vi "OneSensorMagazineLogic.vi"(5 "Intake Side Sensor":bool, 6 "Outtake Button":bool, 7 "Intake Toggle":bool) -> (0 "Intake Pistons":bool, 1 "Kicker Motors":dbl, 2 "Magazine Motors":dbl, 3 "Intake Motors":dbl)   [LabVIEW 2020]
uses:
  MagazineControl.ctl
  OneSensorMagazineLogic.ctl
  TitanLib/Lib/TitanLib.lvlib
panel:
  in  "Initial State":T1
  out "Current State":T2
  in  "Kicker Power":dbl=0.5
  in  "Magazine Power":dbl=1.0
  in  "Input Power":dbl=1.0
  # "Inputs"
  # "Power Levels"
  # "Outputs"
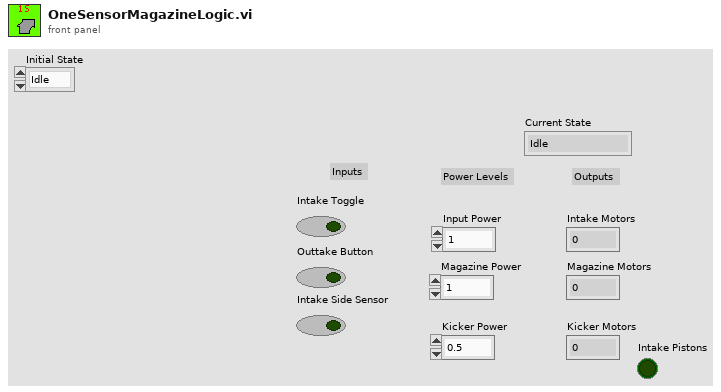
[diagram p1: front panel]
types:
  T1 = typedef "OneSensorMagazineLogic.ctl" = enum16{"Idle", "Intaking", "One Ball", "One Ball Intake", "Two Balls", "Outtake"}
  T2 = typedef "MagazineControl.ctl" = enum16{"Idle", "Intaking", "Outtake", "One Ball", "One Ball Intake", "One Ball Outtake", "Two Balls", "Two Ball Outtake"}
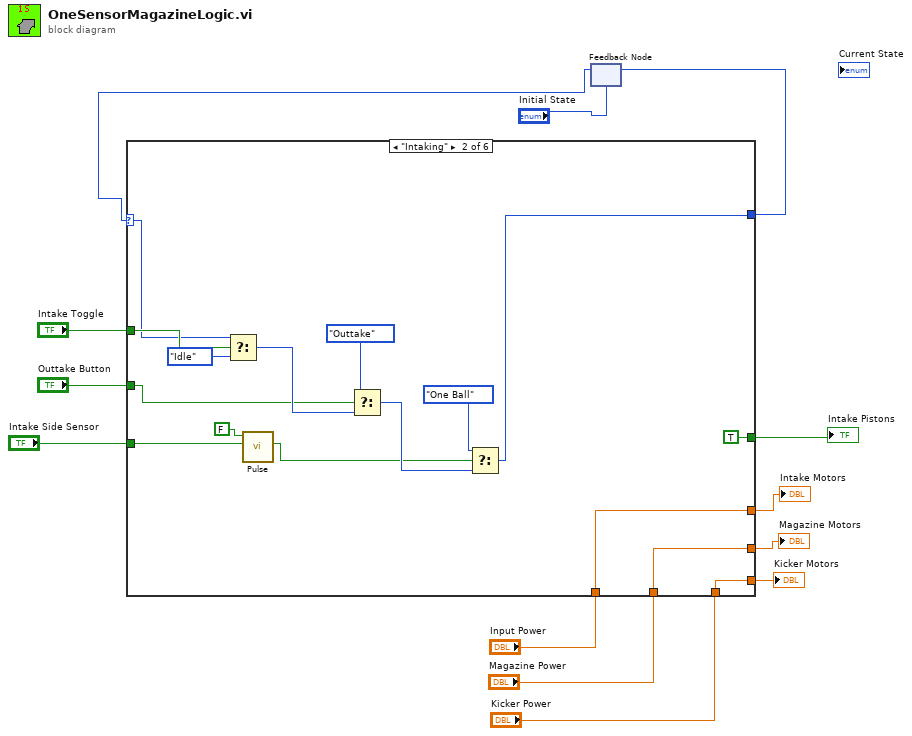
[diagram p0: block diagram]
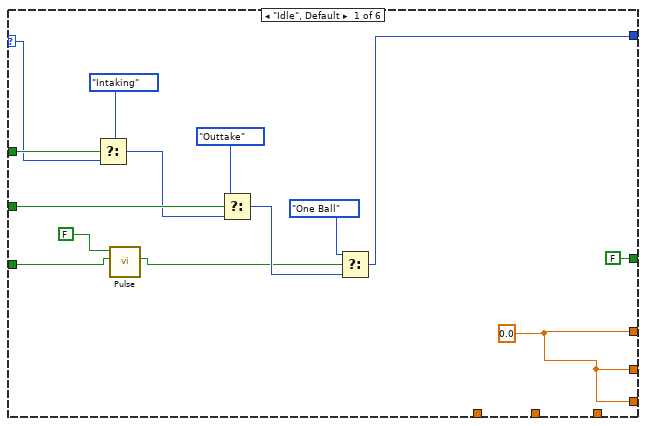
[diagram p2: hidden frame]
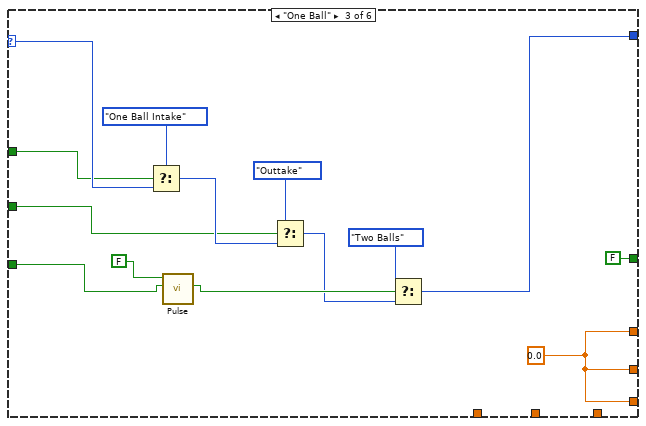
[diagram p3: hidden frame]
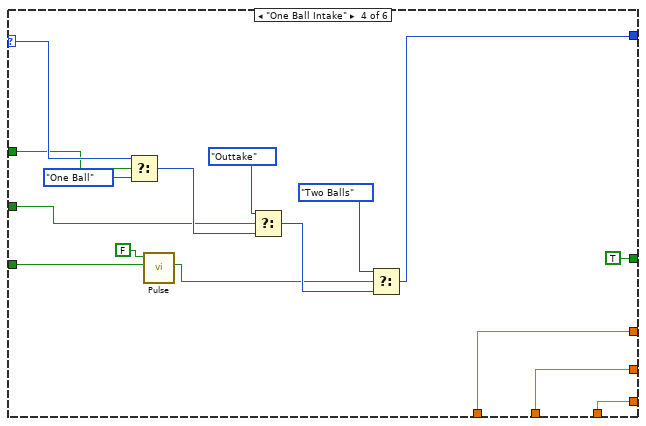
[diagram p4: hidden frame]
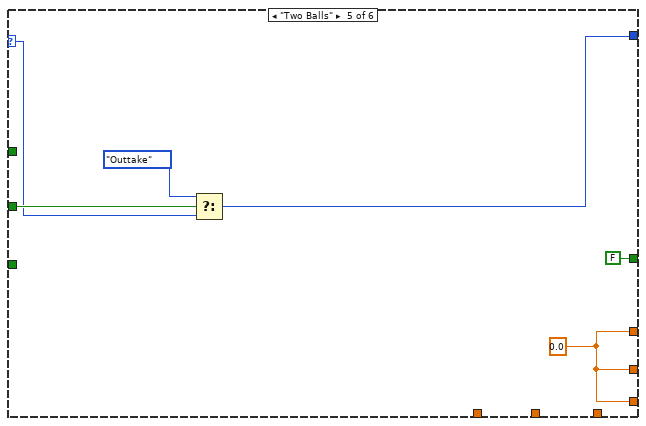
[diagram p5: hidden frame]
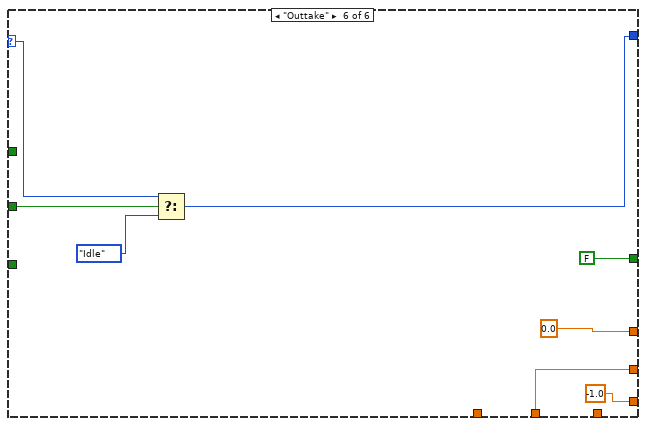
[diagram p6: hidden frame]
diagram:
  n1 = feedback #1("Initial State") -> (w2:T1)
  n2 = case shown="\"Intaking\"" w2 {
    selector: w2 -> [w18 w39 w51 w67 w78 w82]
    tunnel: "Intake Toggle" -> [w27 w41 w50 w66 _ _]
    tunnel: "Outtake Button" -> [w26 w40 w52 w68 w79 w87]
    tunnel: "Intake Side Sensor" -> [w22 w35 w53 w69 _ _]
    tunnel: [w20 w38 w49 w65 w77 0.0 ("Input Power")] -> w8
    tunnel: "Input Power" -> [_ w38 _ w65 _ _]
    tunnel: [w20 w37 w49 w64 w77 w84] -> w10
    tunnel: "Magazine Power" -> [_ w37 _ w64 _ w84]
    tunnel: [w20 w33 w49 w63 w77 -1.0 ("Kicker Motors")] -> w12
    tunnel: "Kicker Power" -> [_ w33 _ w63 _ _]
    tunnel: [FALSE ("Intake Pistons") TRUE ("Intake Pistons") FALSE ("Intake Pistons") TRUE ("Intake Pistons") FALSE ("Intake Pistons") FALSE ("Intake Pistons")] -> w4
    tunnel: [w14 w28 w44 w61 w75 w80] -> w1
    frame "Idle", Default {
      w20 = 0.0 ("Input Power")
      n3 = Select(t=OneSensorMagazineLogic."Intaking", s=w27, f=w18) -> (s? t:f=w25:T1)
      n4 = call "Pulse.vi"("Input"=w22, "Rising Edge?"=FALSE) -> ("Output"=w23:bool)  [unwired: 9 in]
      n5 = Select(t=OneSensorMagazineLogic."Outtake", s=w26, f=w25) -> (s? t:f=w24:T1)
      n6 = Select(t=OneSensorMagazineLogic."One Ball", s=w23, f=w24) -> (s? t:f=w14:T1)
    }
    frame "Intaking" {
      n7 = Select(t=w39, s=w41, f=OneSensorMagazineLogic."Idle") -> (s? t:f=w42:T1)
      n8 = call "Pulse.vi"("Input"=w35, "Rising Edge?"=FALSE) -> ("Output"=w36:bool)  [unwired: 9 in]
      n9 = Select(t=OneSensorMagazineLogic."Outtake", s=w40, f=w42) -> (s? t:f=w43:T1)
      n10 = Select(t=OneSensorMagazineLogic."One Ball", s=w36, f=w43) -> (s? t:f=w28:T1)
    }
    frame "One Ball" {
      w49 = 0.0 ("Input Power")
      n11 = Select(t=OneSensorMagazineLogic."One Ball Intake", s=w50, f=w51) -> (s? t:f=w55:T1)
      n12 = call "Pulse.vi"("Input"=w53, "Rising Edge?"=FALSE) -> ("Output"=w57:bool)  [unwired: 9 in]
      n13 = Select(t=OneSensorMagazineLogic."Outtake", s=w52, f=w55) -> (s? t:f=w56:T1)
      n14 = Select(t=OneSensorMagazineLogic."Two Balls", s=w57, f=w56) -> (s? t:f=w44:T1)
    }
    frame "One Ball Intake" {
      n15 = Select(t=w67, s=w66, f=OneSensorMagazineLogic."One Ball") -> (s? t:f=w72:T1)
      n16 = call "Pulse.vi"("Input"=w69, "Rising Edge?"=FALSE) -> ("Output"=w71:bool)  [unwired: 9 in]
      n17 = Select(t=OneSensorMagazineLogic."Outtake", s=w68, f=w72) -> (s? t:f=w73:T1)
      n18 = Select(t=OneSensorMagazineLogic."Two Balls", s=w71, f=w73) -> (s? t:f=w61:T1)
    }
    frame "Two Balls" {
      w77 = 0.0 ("Input Power")
      n19 = Select(t=OneSensorMagazineLogic."Outtake", s=w79, f=w78) -> (s? t:f=w75:T1)
    }
    frame "Outtake" {
      n20 = Select(t=w82, s=w87, f=OneSensorMagazineLogic."Idle") -> (s? t:f=w80:T1)
    }
  }
  "Intake Motors" <- w8
  "Magazine Motors" <- w10
  "Kicker Motors" <- w12
  "Intake Pistons" <- w4
  n21 = feedback-in #1(w1) -> ()
